vi "WiFi lab coordinator Transparent.vi"() -> ()   [LabVIEW 2017]
uses:
  WiFi API Frame Type.ctl
  WiFi API Frame.ctl
  VISA resource XBee.vi
  <vilib>/Utility/file.llb/Write Delimited Spreadsheet (string).vi
panel:
  in  "stop":bool
  in  "Response":string
  in  "Control string":string
  in  "Start session":bool
  in  "Destination port (hex)":u16=9750 step=1 format="%04x"
  in  "Source port (hex)":u16=2000 step=1 format="%04x"
  out "Array":cluster{"Source IP":u8[], "RF data":string}[](array[cluster])
  out "string":string
  out "Frame Type":T1 items=["Frame Error"=254, "Device Response Status"=186, "Device Request"=185, "Send Data Response"=184, "RX Packet IPv4"=176, "Zigbee Remote AT Command Response"=151, "Explicit Zigbee Receive Packet"=145, "Zigbee Receive Packet"=144, "I/O Sample Rx Indicator"=143, "Zigbee TX Status"=139, "Modem Status"=138, "Transmit Status"=137, "AT Command Response"=136, "Remote Command Response"=135, "Rx Packet"=128, "Device Response"=42, "Send Data Request"=40, "TX Request IPv4"=32, "Zigbee Remote AT Command"=23, "Zigbee Explicit Transmit Packet"=17, "Zigbee Transmit Packet"=16, "AT Command "=8, "Remote AT Command Request"=7, "TX Request"=0]
  # "Session Configuration"
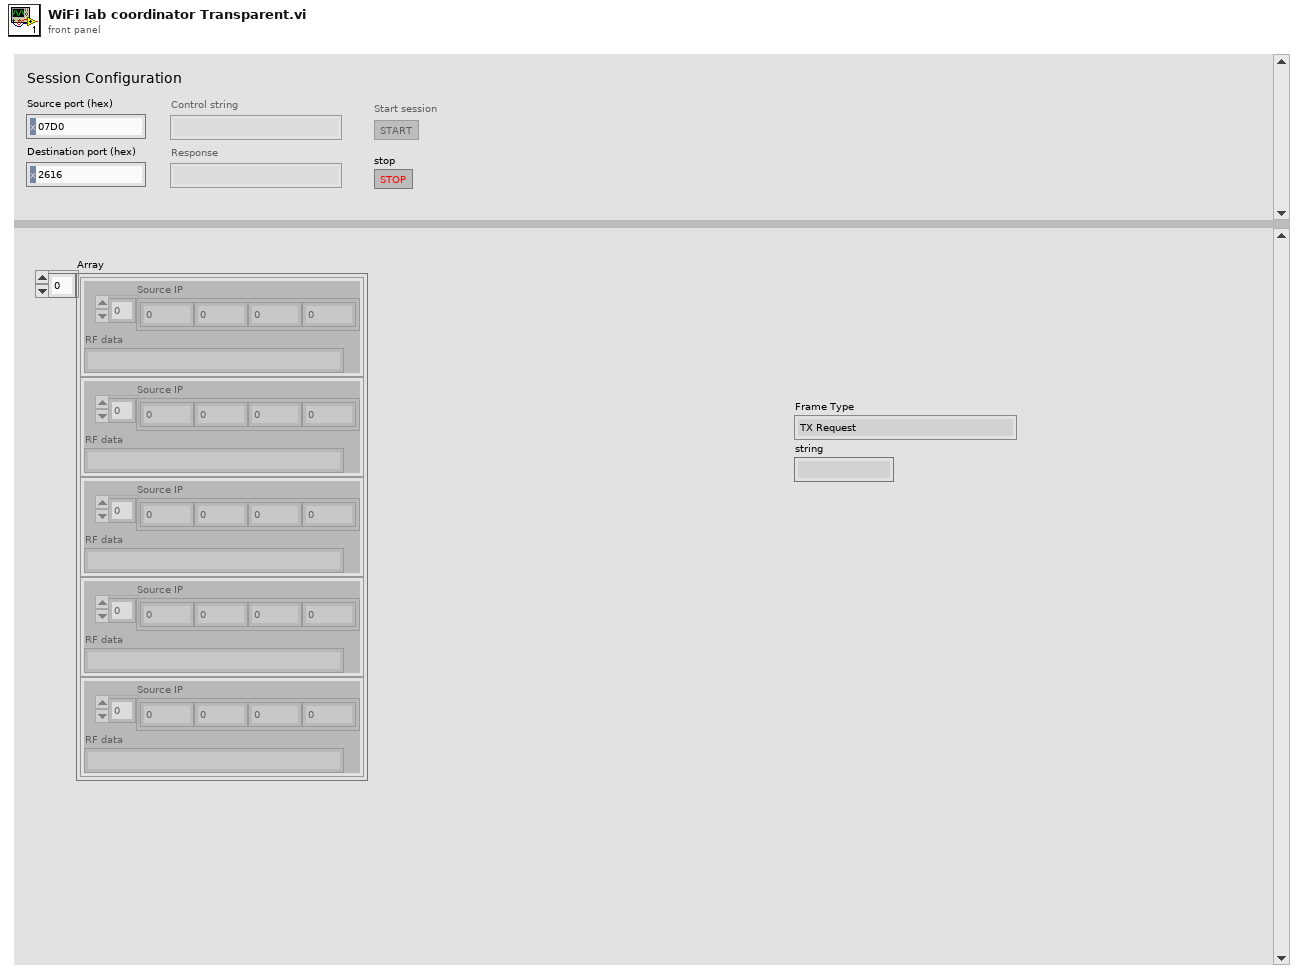
[diagram p1: front panel]
types:
  T1 = typedef "WiFi API Frame Type.ctl" = u8
  T2 = typedef "WiFi API Frame.ctl" = cluster{"Length":u16, "Frame Type":T1, "Payload":u8[], "Checksum":u8}
  T3 = enum8{"Enabled", "Disabled", "Disabled and Grayed Out"}
  T4 = typedef "Protocol enum.ctl" = enum8{"UDP", "TCP"}
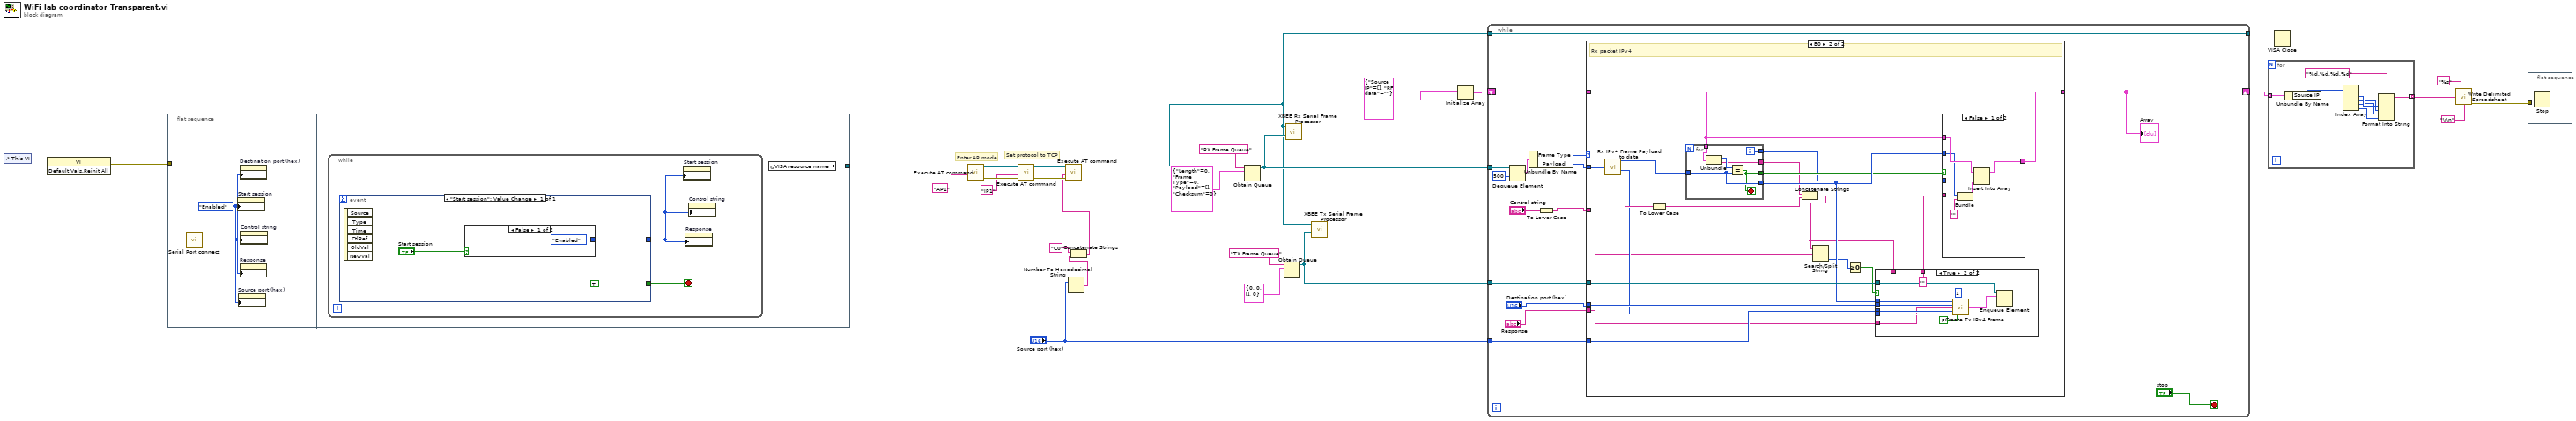
[diagram p0: block diagram]
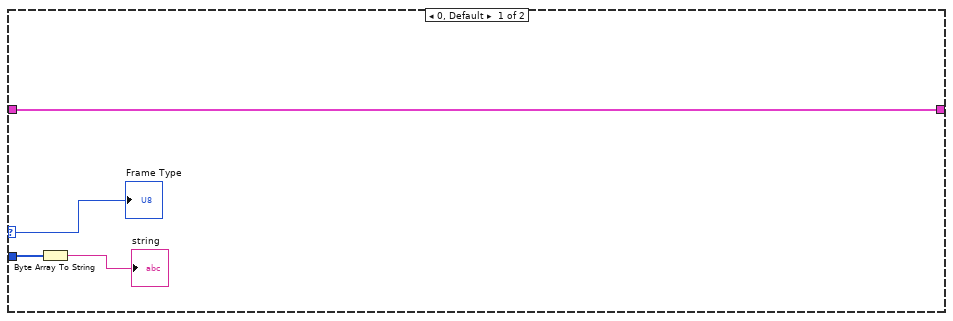
[diagram p2: hidden frame]
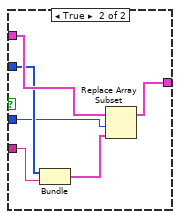
[diagram p4: hidden frame]
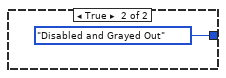
[diagram p5: hidden frame]
diagram:
  # "Set protocol to TCP"
  # "Enter AP mode"
  n1 = control-ref of="This VI"() -> (w13:refnum<vi>)
  n2 = invoke class="VI" method="Default Vals.Reinit All"(reference=w13) -> (error out=w28:errorcluster)  [unwired: 2 in, 2 out]
  n3 = flat-sequence {
    tunnel: w28 -> [_]
    tunnel: [w30] -> w14
    frame #0 {
      w29 = T3."Enabled" ("Disabled")
      n4 = call "Serial Port connect.vi"() -> ()  [unwired: 3 in]
      n5 = property on="Start session" class="Bool"("DisabledEnum"=w29) -> ()  [unwired: 2 in, 2 out]
      n6 = property on="Source port (hex)" class="DigNum (strict)"("DisabledEnum"=w29) -> ()  [unwired: 2 in, 2 out]
      n7 = property on="Destination port (hex)" class="DigNum (strict)"("DisabledEnum"=w29) -> ()  [unwired: 2 in, 2 out]
      n8 = property on="Response" class="Str"("DisabledEnum"=w29) -> ()  [unwired: 2 in, 2 out]
      n9 = property on="Control string" class="Str"("DisabledEnum"=w29) -> ()  [unwired: 2 in, 2 out]
    }
    frame #1 {
      n10 = while {
        stop <- w32 stop-if-true
        n11 = event shown="[0] \"Start session\": Value Change" {
          selector: _ -> [_]
          dyn-events: _ -> [_]
          timeout: _ -> [_]
          tunnel: [w35] -> w31
          tunnel: [TRUE] -> w32
          event "Start session": Value Change {
            n12 = event-data() -> ()  [unwired: 1 in, 6 out]
            n13 = case shown="False" "Start session" {
              tunnel: [T3."Enabled" ("Disabled") T3."Disabled and Grayed Out" ("Disabled")] -> w35
              frame False {
              }
              frame True {
              }
            }
          }
        }
        n14 = property on="Start session" class="Bool"("DisabledEnum"=w31) -> ()  [unwired: 2 in, 2 out]
        n15 = property on="Response" class="Str"("DisabledEnum"=w31) -> ()  [unwired: 2 in, 2 out]
        n16 = property on="Control string" class="Str"("DisabledEnum"=w31) -> ()  [unwired: 2 in, 2 out]
      }
      n17 = global read "VISA resource XBee.vi" "VISA resource name"() -> (w30:refnum<visa-resource-name>)
    }
  }
  n18 = call "Execute AT command.vi"("AT Command"="AP1", "VISA resource in"=w14) -> ("error out"=w17:errorcluster, "VISA resource out"=w18:refnum<visa-resource-name>)  [unwired: 6 in, 1 out]
  n19 = call "Execute AT command.vi"("error in (no error)"=w17, "AT Command"="IP1", "VISA resource in"=w18) -> ("error out"=w11:errorcluster, "VISA resource out"=w12:refnum<visa-resource-name>)  [unwired: 5 in, 1 out]
  n20 = Number To Hexadecimal String(2:"Source port (hex)") -> (0:w6:string)  [unwired: 1 in]
  n21 = Concatenate Strings("C0" ("AT Command"), w6) -> (w8:string)
  n22 = call "Execute AT command.vi"("error in (no error)"=w11, "AT Command"=w8, "VISA resource in"=w12) -> ("VISA resource out"=w10:refnum<visa-resource-name>)  [unwired: 5 in, 2 out]
  n23 = Obtain Queue(name (unnamed)="RX Frame Queue", element data type=T2 {"Length"=0, "Frame Type"=0, "Payload"=[], "Checksum"=0} ("API Frame")) -> (queue out=w23:refnum<queue>)  [unwired: 3 in, 2 out]
  n24 = Obtain Queue(name (unnamed)="TX Frame Queue", element data type=T2 {"Length"=0, "Frame Type"=0, "Payload"=[], "Checksum"=0} ("API Frame")) -> (queue out=w20:refnum<queue>)  [unwired: 3 in, 2 out]
  n25 = call "XBEE Rx Serial Frame Processor.vi"("RX Frame Queue"=w23, "VISA Serial Port"=w10) -> ()  [unwired: 8 in, 2 out]
  n26 = call "XBEE Tx Serial Frame Processor.vi"("TX Frame Queue"=w20, "VISA Serial Port"=w10) -> ()  [unwired: 8 in, 2 out]
  n27 = Initialize Array(cluster{"Source IP":u8[], "RF data":string} {"Source IP"=[], "RF data"=""}) -> (w22:cluster{"Source IP":u8[], "RF data":string}[])  [unwired: 1 in]
  n28 = while {
    tunnel: w23 -> [w52]
    shift-right: [w38] -> w5
    shift-left: w22 -> [w48]
    tunnel: w20 -> [w47]
    tunnel: w10 -> [w42]
    tunnel: [w42] -> w19
    tunnel: "Source port (hex)" -> [w40]
    stop <- "stop" stop-if-true
    n29 = Dequeue Element(queue=w52, timeout in ms (-1)=500) -> (element=w51:T2)  [unwired: 1 in, 3 out]
    n30 = Unbundle By Name(w51) -> ("Frame Type"=w50:T1, "Payload"=w49:u8[])
    n31 = To Lower Case(string="Control string") -> (all lower case string=w45:string)
    n32 = case shown="B0" w50 {
      selector: w50 -> [w55 _]
      tunnel: w49 -> [w54 w76]
      tunnel: w48 -> [w56 w74]
      tunnel: w45 -> [_ w63]
      tunnel: w47 -> [_ w75]
      tunnel: "Destination port (hex)" -> [_ w73]
      tunnel: "Response" -> [_ w57]
      tunnel: w40 -> [_ w72]
      tunnel: [w56 w71] -> w38
      frame 0, Default {
        n33 = Byte Array To String(unsigned byte array=w54) -> (string=→"string":string)
        "Frame Type" <- w55
      }
      frame 176 {
        # "Rx packet IPv4"
        n34 = call "Rx IPv4 Frame Payload to data.vi"("Payload array"=w76) -> ("Source IP"=w69:u8[], "Protocol"=w68:T4, "RF data"=w70:string)  [unwired: 10 in, 2 out]
        n35 = To Lower Case(string=w70) -> (all lower case string=w64:string)
        n36 = for {
          tunnel: w69 -> [w104]
          tunnel: [w103] -> w66
          tunnel: w74 -> [w101] mode=indexing
          tunnel: [w104] -> w67
          tunnel: [w102] -> w58
          tunnel: [w99] -> w65
          i -> [w102]
          stop <- w103 stop-if-true
          n37 = Unbundle(w101) -> ("Source IP"=w100:u8[], "RF data"=w99:string)
          n38 = Equal?(x=w100, y=w104) -> (x = y?=w103:bool)
        }
        n39 = Concatenate Strings(w65, w64) -> (w60:string)
        n40 = Search/Split String(string=w60, search string/char (-)=w63) -> (offset of match=w61:i32)  [unwired: 1 in, 2 out]
        n41 = Greater Or Equal To 0?(x=w61) -> (x >= 0?=w62:bool)
        n42 = case shown="True" w62 {
          tunnel: w75 -> [_ w87]
          tunnel: w73 -> [_ w86]
          tunnel: w72 -> [_ w85]
          tunnel: w68 -> [_ w84]
          tunnel: w67 -> [_ w80]
          tunnel: w60 -> [w77 _]
          tunnel: [w77 ""] -> w59
          tunnel: w57 -> [_ w78]
          frame False {
          }
          frame True {
            n43 = call "Create Tx IPv4 Frame.vi"("Destination IP"=w80, "Frame ID"=u8 1, "Destination port"=w86, "RF data"=w78, "Source port"=w85, "Protocol"=w84, "Transmit options bitfield"=FALSE) -> ("TX IPv4 Frame"=w81:T2)  [unwired: 8 in]
            n44 = Enqueue Element(queue=w87, element=w81) -> ()  [unwired: 2 in, 3 out]
          }
        }
        n45 = case shown="False" w66 {
          tunnel: [w91 w97] -> w71
          tunnel: w74 -> [w92 w98]
          tunnel: w67 -> [w90 w96]
          tunnel: w59 -> [_ w95]
          tunnel: w58 -> [_ w93]
          frame False {
            n46 = Bundle("Source IP"=w90, "") -> (w89:cluster{"Source IP":u8[], string})  [unwired: 1 in]
            n47 = Insert Into Array(array=w92, new element=w89) -> (w91:cluster{"Source IP":u8[], "RF data":string}[])  [unwired: 1 in]
          }
          frame True {
            n48 = Bundle("Source IP"=w96, w95) -> (w94:cluster{"Source IP":u8[], string})  [unwired: 1 in]
            n49 = Replace Array Subset(array=w98, new element=w94, index=w93) -> (w97:cluster{"Source IP":u8[], "RF data":string}[])
          }
        }
      }
    }
    "Array" <- w38
  }
  n50 = for {
    tunnel: w5 -> [w112] mode=indexing
    tunnel: [w105] -> w3 mode=indexing
    n51 = Unbundle By Name(w112) -> ("Source IP"=w110:u8[])
    n52 = Index Array(array=w110) -> (element #1=w109:u8, element #2=w108:u8, element #3=w107:u8, element #4=w106:u8)  [unwired: 4 in]
    n53 = Format Into String(format string="%d.%d.%d.%d", w109, w108, w107, w106) -> (resulting string=w105:string)  [unwired: 2 in, 1 out]
  }
  n54 = VISA Close(VISA resource name=w19) -> ()  [unwired: 1 in, 1 out]
  n55 = call-poly <vilib>:"Write Delimited Spreadsheet.vi"("format (%s)"="%s" ("format (%.3f)"), "1D data"=w3, "delimiter (\\t)"="\r\n") -> ("error out"=w1:errorcluster)  [unwired: 11 in, 1 out]
  n56 = flat-sequence {
    tunnel: w1 -> [_]
    frame #0 {
      n57 = Stop() -> ()  [unwired: 1 in]
    }
  }
